vi "to-matlab3-UI.vi"() -> ()   [LabVIEW 2018]
uses:
  <extravilib>/ChannelInstances/Stream-u32.lvlib
  <extravilib>/ChannelInstances/Stream-a[.](wfm(dbl)).lvlib
  <vilib>/DAQmx/create/channels.llb/DAQmx Create Channel (AI-Voltage-Basic).vi
  <vilib>/platform/TimedLoop/XDataNode/XDataNode.xnode
  <vilib>/Platform/TimedLoop/XDataNode/nitl_modes.ctl
  <vilib>/Platform/TimedLoop/XDataNode/XDNodeRunTimeDep.lvlib
  <vilib>/Platform/TimedLoop/XDataNode/wakeup.ctl
  <vilib>/Platform/TimedLoop/XDataNode/timing_clust.ctl
  <vilib>/DAQmx/read.llb/DAQmx Read (Counter U32 1Chan 1Samp).vi
  <vilib>/DAQmx/configure/timing.llb/DAQmx Timing (Sample Clock).vi
  <vilib>/DAQmx/read.llb/DAQmx Read (Analog 1D Wfm NChan NSamp).vi
  <vilib>/DAQmx/create/channels.llb/DAQmx Create Channel (CI-Count Edges).vi
panel:
  in  "Reset Button":bool
  in  "Start Button":bool
  in  "Stop Button":bool
  in  "Settings Button":bool
  in  "Radio Buttons - Customizable":T1(radio)
  out "System Tab":T2(tab)
  out "All Graphs":dynamicdata(graph) caption="Waveform Chart - dark"
  in  "Brake Torque scale":dbl=1.0
  in  "Batterycurrent scale":dbl=25.0
  in  "Batteryvoltage scale":dbl=9.97
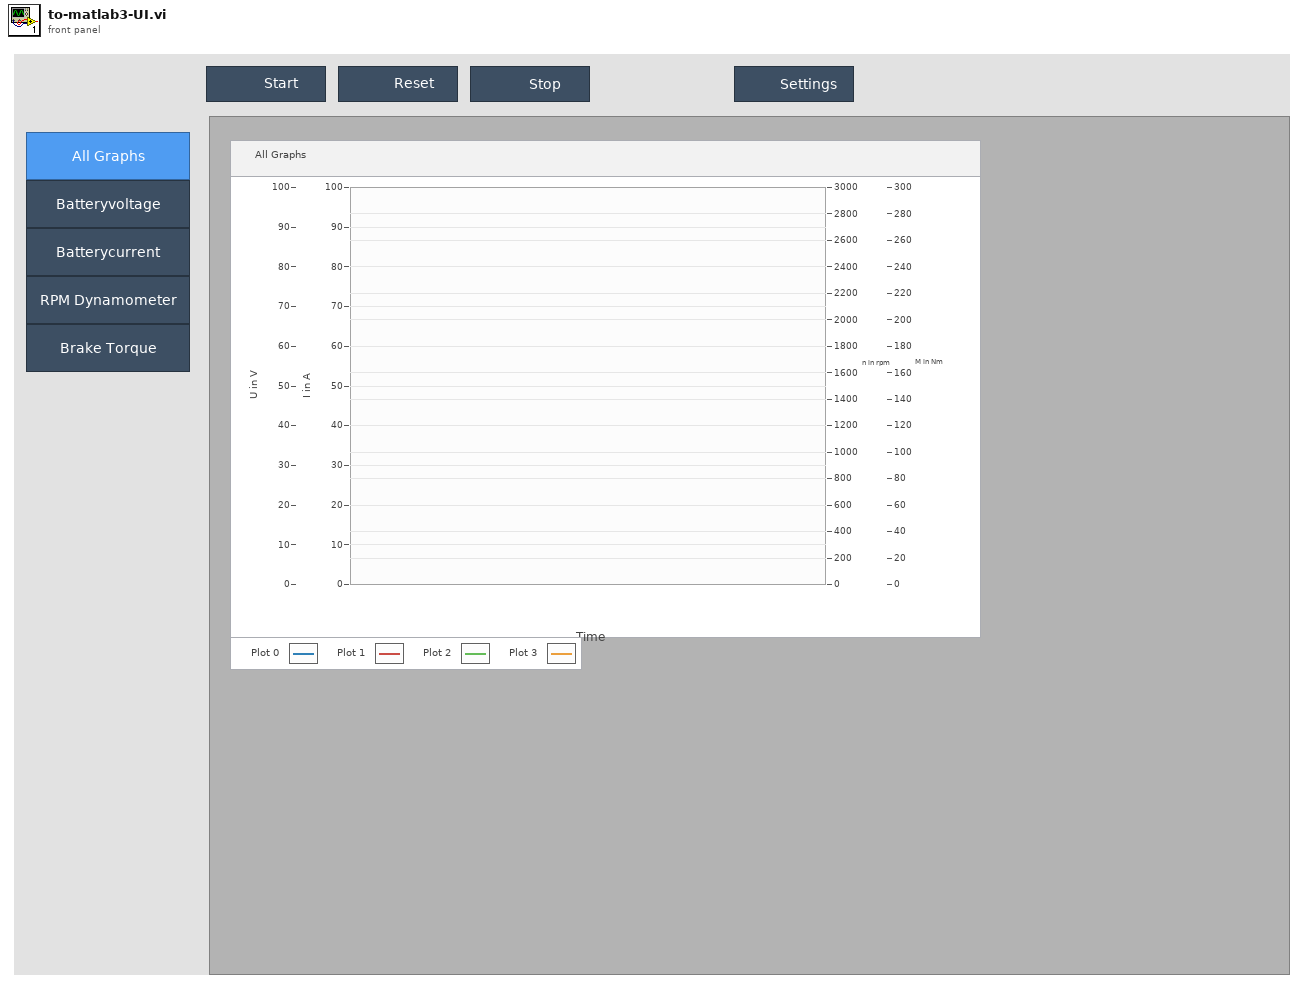
[diagram p1: front panel]
types:
  T1 = enum32{"Standard Button", "Standard Button 2", "Standard Button 3", "Radio Selection 4", "Radio Selection 5"}
  T2 = enum32{"allgraphs-page", "u_batt-page", "i_batt-page", "rpm-page", "mbrems-page", "settings-page"}
  T3 = typedef "XDNodeRunTimeDep.lvlib/timing_clust.ctl" = cluster{"Expected End [f-1]":u64, "Actual End [f-1]":u64, "Finished Late? [f-1]":bool, "Expected End [i-1]":u64, "Actual End [i-1]":u64, "Finished Late? [i-1]":bool, "Expected Start [i]":u64, "Actual Start [i]":u64, "Expected Start [f]":u64, "Actual Start [f]":u64, "Source Name":string, "Structure Name":string, "Period":i64, "Deadline":i64, "Offset":i64, "Start":i64, "Priority":i32, "Timeout":i32, "Mode":T4, "Wakeup Reason":T5, "Error":errorcluster, "Source Type":string, "Secondary Source Type":string, "Global End Time":u64, "Global Start Time":u64, "Frame Duration":u64, "Iteration Duration":u64, "Assigned CPU":i32, "I/O Scan Engine Mode":u32}
  T4 = typedef "XDNodeRunTimeDep.lvlib/nitl_modes.ctl" = enum32{"No Change", "Process missed periods, maintain original phase", "Discard missed periods, maintain original phase", "Process missed periods, ignore original phase", "Discard missed periods, ignore original phase"}
  T5 = typedef "XDNodeRunTimeDep.lvlib/wakeup.ctl" = enum32{"Normal", "Aborted", "Asynchronous wakeup", "Timing source error", "Timed loop error", "Timeout"}
  T6 = typedef "Stream-u32.lvlib/)Channel.ctl" = refnum<queue>
  T7 = typedef "Stream-a[.](wfm(dbl)).lvlib/)Channel.ctl" = refnum<queue>
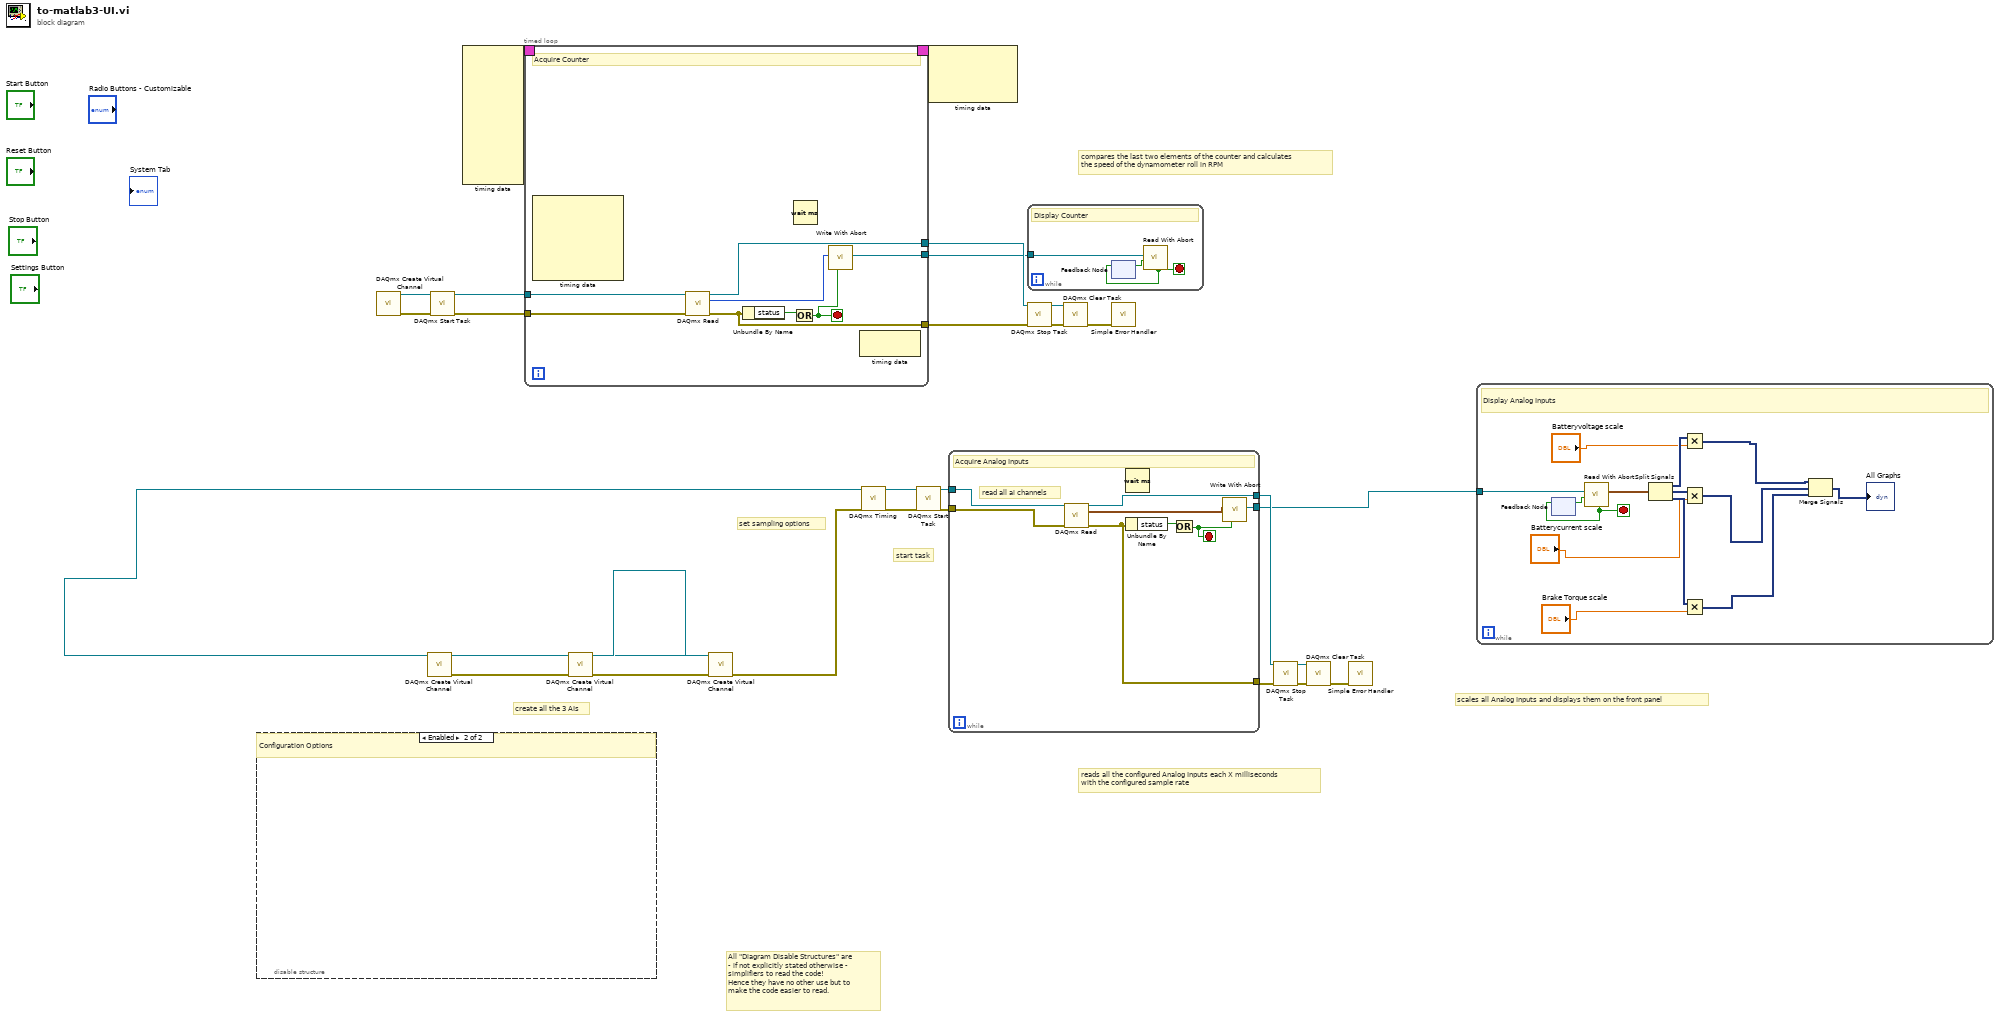
[diagram p0: block diagram]
diagram:
  # "scales all Analog Inputs and displays them on the front panel"
  # "reads all the configured Analog Inputs each X milliseconds\nwith the configured sample rate"
  # "compares the last two elements of the counter and calculates\nthe speed of the dynamometer roll in RPM"
  # "All \"Diagram Disable Structures\" are \n- if not explicitly stated otherwise - \nsimplifiers to read the code!\nHence they have no other use but to \nmake the code easier to read."
  # "start task"
  # "set sampling options"
  # "create all the 3 AIs"
  n1 = disable-structure shown="Enabled" {
    frame Disabled {
    }
    frame Enabled {
      # "Configuration Options"
    }
  }
  n2 = call-poly <vilib>:"DAQmx Create Virtual Channel.vi"() -> ("task out"=w43:refnum<k21>, "counter"=w5:tag, "name to assign"=w4:string, "error out"=w42:errorcluster)  [unwired: 12 in]
  n3 = call-poly <vilib>:"DAQmx Create Virtual Channel.vi"() -> ("input terminal configuration"=w18:i32, "task out"=w17:refnum<k21>, "physical channels"=w26:tag, "name to assign"=w19:string, "error out"=w16:errorcluster)  [unwired: 11 in]
  n4 = call <vilib>:"DAQmx Start Task.vi"("task/channels in"=w43, "error in"=w42) -> ("task out"=w41:refnum<k21>, "error out"=w40:errorcluster)  [unwired: 12 in]
  n5 = node-c288() -> (w3:T3)  [unwired: 10 in]
  n6 = timed-loop {
    tunnel: w41 -> [w54]
    tunnel: w40 -> [w53]
    tunnel: [w50] -> w37
    tunnel: [w52] -> w36
    tunnel: [w46] -> w34
    timing: w3 -> [_]
    timing-out: [_] -> w2
    stop <- w47 stop-if-true
    # "Acquire Counter"
    n7 = node-c288() -> (w44:i64)  [unwired: 1 in, 5 out]
    n8 = call-poly <vilib>:"DAQmx Read.vi"("task/channels in"=w54, "error in"=w53) -> ("task out"=w52:refnum<k21>, "data"=w48:u32, "error out"=w50:errorcluster)  [unwired: 11 in]
    n9 = Unbundle By Name(w50) -> ("status"=w49:bool)
    n10 = Or(x=w49) -> (y=w51:bool, x .or. y?=w47:bool)
    n11 = Wait (ms)() -> (milliseconds to wait=w45:u32)  [unwired: 1 out]
    n12 = call <extravilib>:"Write With Abort.vi"("abort"=w47, "element"=w48) -> ("channel"=w46:T6)  [unwired: 6 in, 3 out]
    n13 = node-c288() -> ()  [unwired: 1 in, 1 out]
  }
  n14 = call-poly <vilib>:"DAQmx Create Virtual Channel.vi"("task in"=w17, "error in"=w16) -> ("input terminal configuration"=w9:i32, "task out"=w15:refnum<k21>, "physical channels"=w11:tag, "name to assign"=w10:string, "error out"=w13:errorcluster)  [unwired: 9 in]
  n15 = call-poly <vilib>:"DAQmx Create Virtual Channel.vi"("task in"=w15, "error in"=w13) -> ("input terminal configuration"=w6:i32, "task out"=w14:refnum<k21>, "physical channels"=w8:tag, "name to assign"=w7:string, "error out"=w12:errorcluster)  [unwired: 9 in]
  n16 = call-poly <vilib>:"DAQmx Timing.vi"("task/channels in"=w14, "error in"=w12) -> ("sample mode"=w23:i32, "samples per channel"=w22:i32, "task out"=w30:refnum<k21>, "rate"=w25:dbl, "error out"=w29:errorcluster)  [unwired: 9 in]
  n17 = call <vilib>:"DAQmx Start Task.vi"("task/channels in"=w30, "error in"=w29) -> ("task out"=w21:refnum<k21>, "error out"=w20:errorcluster)  [unwired: 12 in]
  n18 = node-c288(w2) -> (w1:i64)  [unwired: 2 out]
  n19 = while {
    tunnel: w21 -> [w65]
    tunnel: [w63] -> w28
    tunnel: [w64] -> w27
    tunnel: [w59] -> w24
    tunnel: w20 -> [w58]
    stop <- w60 stop-if-true
    # "Acquire Analog Inputs"
    # "read all ai channels"
    n20 = call-poly <vilib>:"DAQmx Read.vi"("task/channels in"=w65, "error in"=w58) -> ("task out"=w64:refnum<k21>, "data"=w61:waveform(dbl)[], "error out"=w63:errorcluster)  [unwired: 11 in]
    n21 = Wait (ms)() -> ()  [unwired: 1 in, 1 out]
    n22 = Unbundle By Name(w63) -> ("status"=w62:bool)
    n23 = Or(x=w62) -> (x .or. y?=w60:bool)  [unwired: 1 in]
    n24 = call <extravilib>:"Write With Abort.vi"("abort"=w60, "element"=w61) -> ("channel"=w59:T7)  [unwired: 6 in, 3 out]
  }
  n25 = while {
    tunnel: w34 -> [w68]
    stop <- w66 stop-if-true
    # "Display Counter"
    n26 = feedback #1() -> (w67:bool)  [unwired: 1 in]
    n27 = call <extravilib>:"Read With Abort.vi"("abort"=w67, "channel"=w68) -> ("aborted?"=w66:bool)  [unwired: 4 in, 5 out]
    n28 = feedback-in #1(w66) -> ()
  }
  n29 = call <vilib>:"DAQmx Stop Task.vi"("task/channels in"=w36, "error in"=w37) -> ("task out"=w35:refnum<k21>, "error out"=w39:errorcluster)  [unwired: 12 in]
  n30 = call <vilib>:"DAQmx Clear Task.vi"("task in"=w35, "error in"=w39) -> ("error out"=w38:errorcluster)  [unwired: 13 in]
  n31 = call <vilib>:"Simple Error Handler.vi"("error in (no error)"=w38) -> ()  [unwired: 4 in, 5 out]
  n32 = call <vilib>:"DAQmx Stop Task.vi"("task/channels in"=w27, "error in"=w28) -> ("task out"=w31:refnum<k21>, "error out"=w33:errorcluster)  [unwired: 12 in]
  n33 = call <vilib>:"DAQmx Clear Task.vi"("task in"=w31, "error in"=w33) -> ("error out"=w32:errorcluster)  [unwired: 13 in]
  n34 = call <vilib>:"Simple Error Handler.vi"("error in (no error)"=w32) -> ()  [unwired: 4 in, 5 out]
  n35 = while {
    tunnel: w24 -> [w82]
    stop <- w81 stop-if-true
    # "Display Analog Inputs"
    n36 = feedback #2() -> (w80:bool)  [unwired: 1 in]
    n37 = call <extravilib>:"Read With Abort.vi"("abort"=w80, "channel"=w82) -> ("element"=w79:waveform(dbl)[], "aborted?"=w81:bool)  [unwired: 4 in, 4 out]
    n38 = feedback-in #2(w81) -> ()
    n39 = Split Signals(w79) -> (w77:dynamicdata, w78:dynamicdata, w76:dynamicdata)  [unwired: 3 in]
    n40 = Multiply(x=w77, y="Batteryvoltage scale") -> (x*y=w71:dynamicdata)
    n41 = Multiply(x=w78, y="Batterycurrent scale") -> (x*y=w70:dynamicdata)
    n42 = Multiply(x=w76, y="Brake Torque scale") -> (x*y=w69:dynamicdata)
    n43 = Merge Signals(w71, w70, w69) -> (→"All Graphs":dynamicdata)
  }
